vi "SetConfig.vi"(8 "error in (no error)":errorcluster, 10 "PARAM":string, 11 "Controlador in":refnum<class "Controlador.lvclass">) -> (0 "error out":errorcluster, 2 "RESP":string, 3 "Controlador out":refnum<class "Controlador.lvclass">)   [LabVIEW 2018, in "Controlador.lvclass"]
uses:
  Controlador.lvclass
  Controlador.lvclass/Controlador.ctl
  <vilib>/Utility/config.llb/Write Key (String).vi
  <vilib>/Utility/config.llb/NI_LVConfig.lvlib
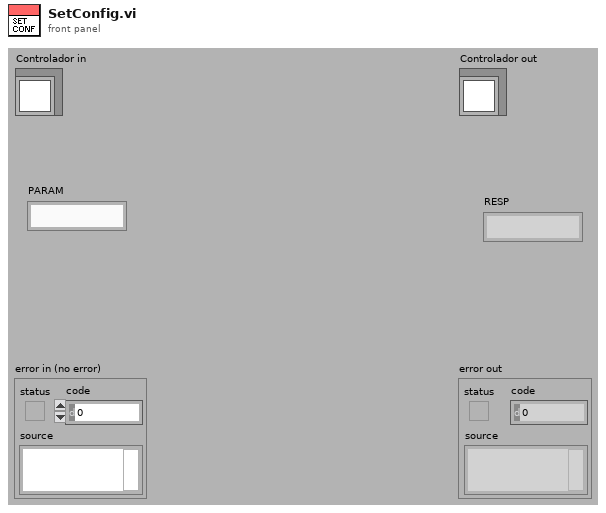
[diagram p1: front panel]
types:
  T1 = typedef "NI_LVConfig.lvlib/Config Data RefNum.ctl" = refnum<k1>
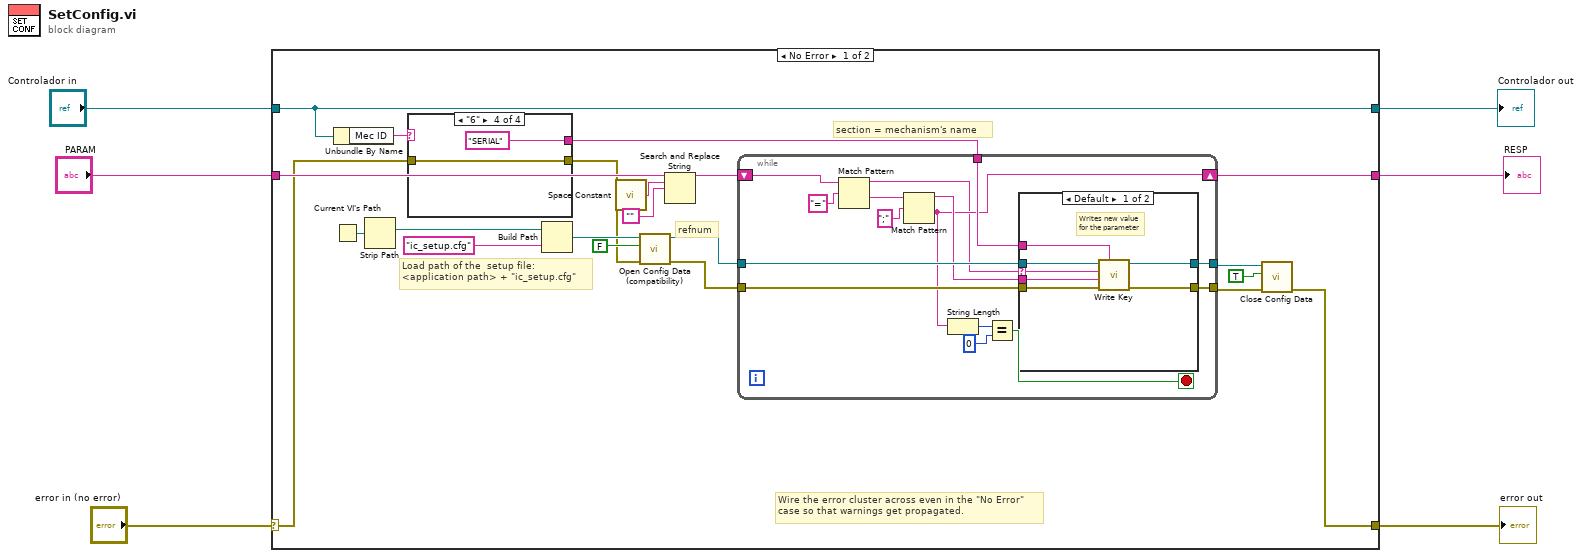
[diagram p0: block diagram]
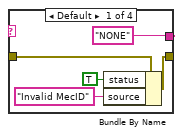
[diagram p2: hidden frame]
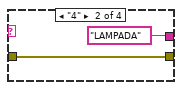
[diagram p3: hidden frame]
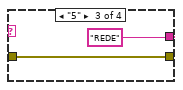
[diagram p4: hidden frame]
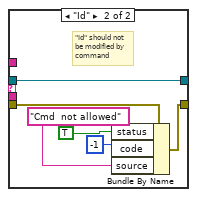
[diagram p5: hidden frame]
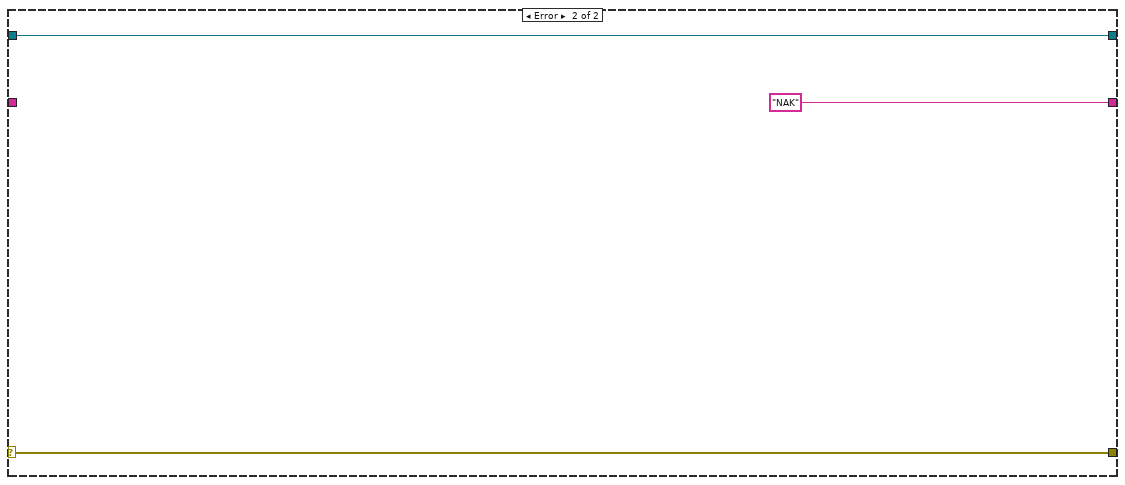
[diagram p6: hidden frame]
diagram:
  n1 = case shown="No Error" "error in (no error)" {
    selector: "error in (no error)" -> [w9 w69]
    tunnel: [w18 w69] -> w3
    tunnel: [w12 w68] -> w4
    tunnel: "Controlador in" -> [w12 w68]
    tunnel: "PARAM" -> [w16 _]
    tunnel: [w7 "NAK" ("result string")] -> w1
    frame No Error {
      # "refnum"
      # "section = mechanism's name"
      # "Load path of the  setup file:\n<application path> + \"ic_setup.cfg\""
      # "Wire the error cluster across even in the \"No Error\"\ncase so that warnings get propagated."
      n2 = Current VI's Path() -> (path=w24:path)
      n3 = Unbundle By Name(w12) -> ("Mec ID"=w11:string)
      n4 = Strip Path(path=w24) -> (stripped path=w25:path)  [unwired: 1 out]
      n5 = case shown="\"6\"" w11 {
        tunnel: ["NONE" "LAMPADA" "REDE" "SERIAL"] -> w10
        tunnel: w9 -> [w31 w33 w35 w37]
        tunnel: [w30 w33 w35 w37] -> w8
        frame Default {
          n6 = Bundle By Name(cluster=w31, "status"=TRUE, "source"="Invalid MecID") -> (w30:errorcluster)
        }
        frame "4" {
        }
        frame "5" {
        }
        frame "6" {
        }
      }
      n7 = Build Path(base path=w25, name or relative path="ic_setup.cfg") -> (appended path=w27:path)
      n8 = call <vilib>:"Space Constant.vi"() -> ("String"=w14:string)
      n9 = call <vilib>:"Open Config Data (compatibility).vi"("error in (no error)"=w8, "create file if necessary (T)"=FALSE ("create file if necessary? (T)"), "configuration file path"=w27) -> ("error out"=w21:errorcluster, "refnum"=w22:T1)  [unwired: 6 in, 1 out]
      n10 = Search and Replace String(input string=w16, search string=w14, replace string="") -> (result string=w15:string)  [unwired: 1 in, 7 out]
      n11 = while {
        tunnel: w22 -> [w53]
        tunnel: w21 -> [w52]
        tunnel: w10 -> [w51]
        shift-right: [w45] -> w7
        shift-left: w15 -> [w50]
        tunnel: [w43] -> w20
        tunnel: [w41] -> w19
        stop <- w40 stop-if-true
        n12 = Match Pattern(string=w50, regular expression="=") -> (before substring=w39:string, after substring=w48:string)  [unwired: 3 out]
        n13 = Match Pattern(string=w48, regular expression=";") -> (before substring=w46:string, after substring=w45:string)  [unwired: 3 out]
        n14 = String Length(string=w45) -> (length=w44:i32)
        n15 = Equal?(x=w44, y=0) -> (x = y?=w40:bool)
        n16 = case shown="Default" w39 {
          selector: w39 -> [w55 _]
          tunnel: w53 -> [w60 w66]
          tunnel: w52 -> [w59 w65]
          tunnel: w51 -> [w54 _]
          tunnel: w46 -> [w58 _]
          tunnel: [w57 w64] -> w43
          tunnel: [w56 w66] -> w41
          frame Default {
            # "Writes new value\nfor the parameter"
            n17 = call-poly <vilib>:"Write Key.vi"("section"=w54, "error in (no error)"=w59, "value"=w58, "key"=w55, "refnum"=w60) -> ("error out"=w57:errorcluster, "refnum out"=w56:T1)  [unwired: 1 in, 4 out]
          }
          frame "Id" {
            # "\"Id\" should not\nbe modified by \ncommand"
            n18 = Bundle By Name(cluster=w65, "status"=TRUE, "code"=-1, "source"="Cmd  not allowed") -> (w64:errorcluster)
          }
        }
      }
      n19 = call <vilib>:"Close Config Data.vi"("error in (no error)"=w20, "write file if changed (T)"=TRUE ("write configuration file? (T)"), "refnum"=w19) -> ("error out"=w18:errorcluster)  [unwired: 8 out]
    }
    frame Error {
    }
  }
  "error out" <- w3
  "Controlador out" <- w4
  "RESP" <- w1
